vi "xijk_combined_file_save.vi"(8 "error in":errorcluster, 10 "queue in":refnum<queue>, 11 "Settings":T1={"search parameters"={"Paths"={"Path: Excitation filters"=path "", "Path: Dicroic filters"=path "", "Path: Emission filters"=path "", "Path reget"=path ""}, "table excitation"=[], "table dicroics"=[], "table emission"=[], "Integers"={"Select result number"=1}, "boolean selector array"=[], "table for calculation automagic"=[]}, "output cluster"={"Booleans"={"Unknown detector"=FALSE, "Dual band filters"=FALSE, "Dual emission by cubes"=FALSE, "FRET"=FALSE}, "Integers"={"Light source"=0, "Number of fluorophores"=0, "Wavelength of laser (nm) 1"=0, "Broadness of laser (nm) 1"=0.0, "Wavelength of laser (nm) 2"=0, "Broadness of laser (nm) 2"=0.0, "Template"=1}, "Doubles"={"Molar extinction 1"=1.0, "Molar extinction 2"=1.0, "Quantum efficiency 1"=1.0, "Quantum efficiency 2"=1.0}}, "output cluster 2"={"Excitation filter 1"=path "", "Dichroic filter 1"=path "", "Emission filter 1"=path "", "Excitation filter 2"=path "", "Dichroic filter 2"=path "", "Emission filter 2"=path "", "Extra em filter 1"=path "", "Extra em filter 2"=path "", "Light source file"=path "", "Fluorophore absorption 1"=path "", "Fluorophore emission 1"=path "", "Fluorophore absorption 2"=path "", "Fluorophore emission 2"=path "", "Detector"=path ""}, "cluster de sortie"={"Excitation filter_x"=[], "Excitation filter_y"=[], "Dichroic filter_x"=[], "Dichroic filter_y"=[], "Emission filter_x"=[], "Emission filter_y"=[], "Excitation filter_x 2"=[], "Excitation filter_y 2"=[], "Dichroic filter_x 2"=[], "Dichroic filter_y 2"=[], "Emission filter_x 2"=[], "Emission filter_y 2"=[], "Extra em filter_x 1"=[], "Extra em filter_y 1"=[], "Extra em filter_x 1"=[], "Extra em filter_y 2"=[], "Light source_x"=[], "Light source_y"=[], "Detector_x"=[], "Detector_y"=[], "Fluorophore absorption_x"=[], "Fluorophore absorption_y"=[], "Fluorophore emission_x"=[], "Fluorophore emission_y"=[], "Fluorophore absorption_x 2"=[], "Fluorophore absorption_y 2"=[], "Fluorophore emission_x 2"=[], "Fluorophore emission_y 2"=[], "laser_x"=[], "laser_y"=[], "laser_x 2"=[], "laser_y 2"=[], "quantum efficiency factor 1"=0.0, "quantum efficiency factor 2"=0.0, "lamp scaling factor"=0.0}, "Xijk output cluster"={"Xijk 111"=0.0, "Xijk 112"=0.0, "Xijk 121"=0.0, "Xijk 122"=0.0, "Xijk 211"=0.0, "Xijk 212"=0.0, "Xijk 221"=0.0, "Xijk 222"=0.0, "Eijk 111"=0.0, "Eijk 112"=0.0, "Eijk 121"=0.0, "Eijk 122"=0.0, "Eijk 211"=0.0, "Eijk 212"=0.0, "Eijk 221"=0.0, "Eijk 222"=0.0}, "GUI configuration"={"axes in"={"min x-axis excitation"=300, "max x-axis excitation"=800, "min x-axis emission"=300, "max x-axis emission"=800, "precision of results"=2}, "plot colors in"={"Lanscape Portrait"=FALSE, "Plot logarithmic"=FALSE, "Ex/Em filters double"=FALSE, "Line colors"=[16734569, 56375, 16711916, 5896447, 16448250, 56375]}}, "references"={"Excitation filter 1 ref"=refnum, "Dichroic filter 1 ref"=refnum, "Emission filter 1 ref"=refnum, "Excitation filter 2 ref"=refnum, "Dichroic filter 2 ref"=refnum, "Emission filter 2 ref"=refnum, "Extra em filter 1 ref"=refnum, "Extra em filter 2 ref"=refnum, "Light source file ref"=refnum, "Fluorophore absorption 1 ref"=refnum, "Fluorophore emission 1 ref"=refnum, "Fluorophore absorption 2 ref"=refnum, "Fluorophore emission 2 ref"=refnum, "Detector ref"=refnum}} {"GUI configuration"."axes in"."precision of results" max=8 step=1}) -> (0 "error out":errorcluster, 2 "queue out":refnum<queue>, 3 "Settings out":T1 {"GUI configuration"."axes in"."precision of results" max=8 step=1})   [LabVIEW 2009, in "xijk_combined_file.lvlib"]
uses:
  xijk_combined_file.lvlib
  Type Def/event.ctl
  Type Def/settings.ctl
  Type Def/search_parameters.ctl
  Type Def/spectra_parameters.ctl
  Type Def/filepath.ctl
  Type Def/spectrum_table_control.ctl
  Type Def/xijk_cluster.ctl
  Type Def/configuration_cluster.ctl
  Type Def/axis_parameters.ctl
  Type Def/color_parameters.ctl
  Type Def/control_references_cluster.ctl
panel:
  # "Dichroic"
  # "Ex/Em filter"
  # "Fluorophore 1"
  # "Fluorophore 2"
  # "Laser /\nextra Em filter"
  # "Dichroic"
  # "Ex/Em filter"
  # "Fluorophore 1"
  # "Fluorophore 2"
  # "Laser /\nextra Em filter"
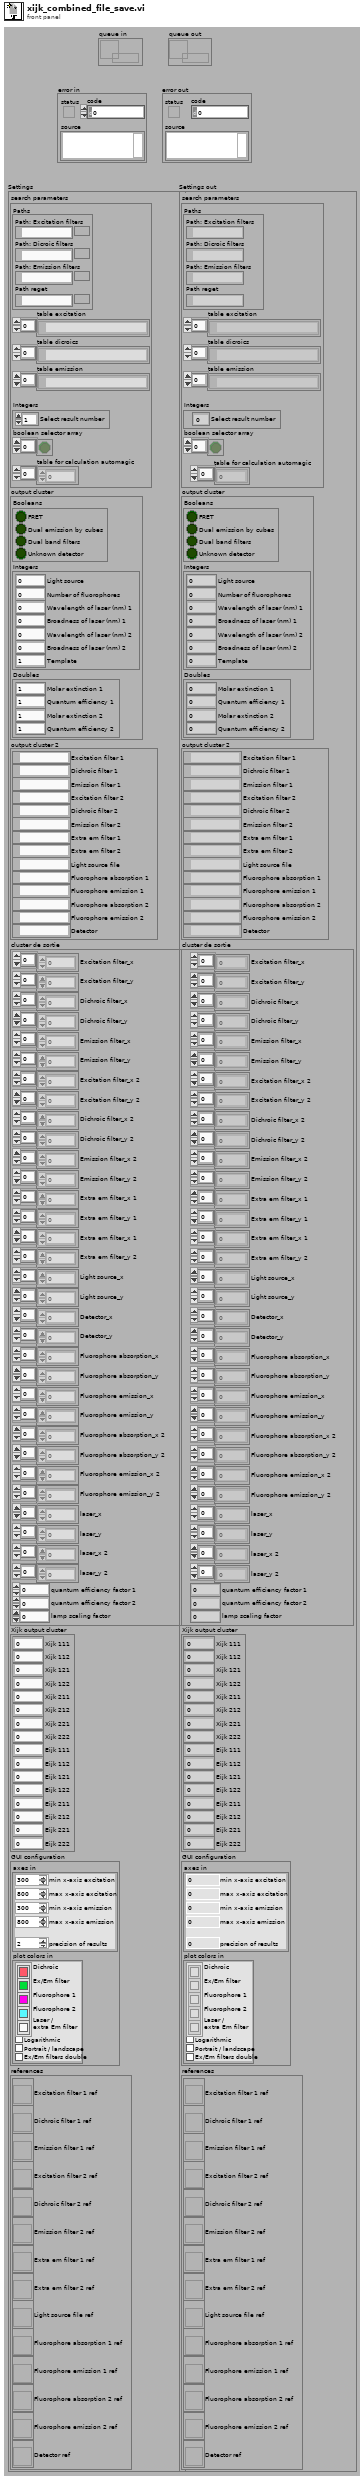
[diagram p1: front panel]
types:
  T1 = typedef "settings.ctl" = cluster{"search parameters":T2, "output cluster":T3, "output cluster 2":T4, "cluster de sortie":T5, "Xijk output cluster":T6, "GUI configuration":T7, "references":T10}
  T2 = typedef "search_parameters.ctl" = cluster{"Paths":cluster{"Path: Excitation filters":path, "Path: Dicroic filters":path, "Path: Emission filters":path, "Path reget":path}, "table excitation":path[], "table dicroics":path[], "table emission":path[], "Integers":cluster{"Select result number":u32}, "boolean selector array":bool[], "table for calculation automagic":i32[]}
  T3 = typedef "spectra_parameters.ctl" = cluster{"Booleans":cluster{"Unknown detector":bool, "Dual band filters":bool, "Dual emission by cubes":bool, "FRET":bool}, "Integers":cluster{"Light source":u16, "Number of fluorophores":u16, "Wavelength of laser (nm) 1":u16, "Broadness of laser (nm) 1":sgl, "Wavelength of laser (nm) 2":u16, "Broadness of laser (nm) 2":sgl, "Template":u16}, "Doubles":cluster{"Molar extinction 1":sgl, "Molar extinction 2":sgl, "Quantum efficiency 1":sgl, "Quantum efficiency 2":sgl}}
  T4 = typedef "filepath.ctl" = cluster{"Excitation filter 1":path, "Dichroic filter 1":path, "Emission filter 1":path, "Excitation filter 2":path, "Dichroic filter 2":path, "Emission filter 2":path, "Extra em filter 1":path, "Extra em filter 2":path, "Light source file":path, "Fluorophore absorption 1":path, "Fluorophore emission 1":path, "Fluorophore absorption 2":path, "Fluorophore emission 2":path, "Detector":path}
  T5 = typedef "spectrum_table_control.ctl" = cluster{"Excitation filter_x":i16[], "Excitation filter_y":sgl[], "Dichroic filter_x":i16[], "Dichroic filter_y":sgl[], "Emission filter_x":i16[], "Emission filter_y":sgl[], "Excitation filter_x 2":i16[], "Excitation filter_y 2":sgl[], "Dichroic filter_x 2":i16[], "Dichroic filter_y 2":sgl[], "Emission filter_x 2":i16[], "Emission filter_y 2":sgl[], "Extra em filter_x 1":i16[], "Extra em filter_y 1":sgl[], "Extra em filter_x 1":i16[], "Extra em filter_y 2":sgl[], "Light source_x":i16[], "Light source_y":sgl[], "Detector_x":i16[], "Detector_y":sgl[], "Fluorophore absorption_x":i16[], "Fluorophore absorption_y":sgl[], "Fluorophore emission_x":i16[], "Fluorophore emission_y":sgl[], "Fluorophore absorption_x 2":i16[], "Fluorophore absorption_y 2":sgl[], "Fluorophore emission_x 2":i16[], "Fluorophore emission_y 2":sgl[], "laser_x":i16[], "laser_y":sgl[], "laser_x 2":i16[], "laser_y 2":sgl[], "quantum efficiency factor 1":sgl, "quantum efficiency factor 2":sgl, "lamp scaling factor":sgl}
  T6 = typedef "xijk_cluster.ctl" = cluster{"Xijk 111":sgl, "Xijk 112":sgl, "Xijk 121":sgl, "Xijk 122":sgl, "Xijk 211":sgl, "Xijk 212":sgl, "Xijk 221":sgl, "Xijk 222":sgl, "Eijk 111":sgl, "Eijk 112":sgl, "Eijk 121":sgl, "Eijk 122":sgl, "Eijk 211":sgl, "Eijk 212":sgl, "Eijk 221":sgl, "Eijk 222":sgl}
  T7 = typedef "configuration_cluster.ctl" = cluster{"axes in":T8, "plot colors in":T9}
  T8 = typedef "axis_parameters.ctl" = cluster{"min x-axis excitation":u16, "max x-axis excitation":u16, "min x-axis emission":u16, "max x-axis emission":u16, "precision of results":u8}
  T9 = typedef "color_parameters.ctl" = cluster{"Lanscape Portrait":bool, "Plot logarithmic":bool, "Ex/Em filters double":bool, "Line colors":u32[]}
  T10 = typedef "control_references_cluster.ctl" = cluster{"Excitation filter 1 ref":refnum<vi>, "Dichroic filter 1 ref":refnum<vi>, "Emission filter 1 ref":refnum<vi>, "Excitation filter 2 ref":refnum<vi>, "Dichroic filter 2 ref":refnum<vi>, "Emission filter 2 ref":refnum<vi>, "Extra em filter 1 ref":refnum<vi>, "Extra em filter 2 ref":refnum<vi>, "Light source file ref":refnum<vi>, "Fluorophore absorption 1 ref":refnum<vi>, "Fluorophore emission 1 ref":refnum<vi>, "Fluorophore absorption 2 ref":refnum<vi>, "Fluorophore emission 2 ref":refnum<vi>, "Detector ref":refnum<vi>}
  T11 = typedef "event.ctl" = enum16{"Initialise parameters", "Initialise paths", "Execute", "Hide detector", "Light source selection", "Get example list", "Set Example", "Change portrait / landscape", "Dual band cube", "Save to file", "Load from file", "Set filepaths to boxes", "1 or 2 fluorophore selection", "Update configurations", "Update template", "Set to personal template", "Calculate other values", "Update filter names", "Shutdown", "Shutdown - hard exit", "Search in filters - set parameters", "Search in filters - search", "Search in filters - get xijk", "Search in filters - reget", "Optimize - Sort table", "Get path from search", "Calculate Xijk", "Get spectra from files", "Create graphs", "Reset variables", "Help - open", "Help - close", "Help - next", "Help - previous", "Help - select menu", "Export data"}
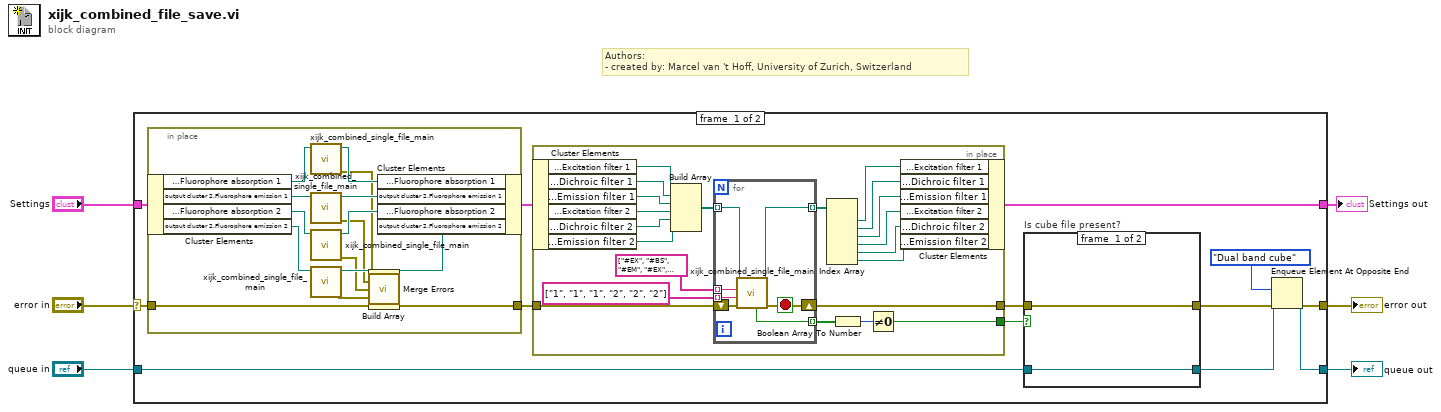
[diagram p0: block diagram]
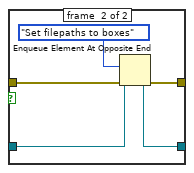
[diagram p2: hidden frame]
diagram:
  # "Authors: \n- created by: Marcel van 't Hoff, University of Zurich, Switzerland"
  n1 = case shown="No Error" "error in" {
    selector: "error in" -> [w10 w72]
    tunnel: [w16 w72] -> w6
    tunnel: "Settings" -> [w11 w71]
    tunnel: [w7 w71] -> w1
    tunnel: [w13 w70] -> w4
    tunnel: "queue in" -> [w18 w70]
    frame #0 {
      n2 = in-place {
        in-place-border: [w50] -> w9
        in-place-border: w10 -> [w49]
        n3 = in-place-cluster #1(w11) -> ("output cluster 2.Fluorophore absorption 1"=w62:path, "output cluster 2.Fluorophore emission 1"=w60:path, "output cluster 2.Fluorophore absorption 2"=w56:path, "output cluster 2.Fluorophore emission 2"=w58:path)
        n4 = call "xijk_combined_single_file_main.vi"("file path in"=w62) -> ("error out"=w51:errorcluster, "file path out"=w61:path)  [unwired: 8 in, 1 out]
        n5 = call "xijk_combined_single_file_main.vi"("file path in"=w60) -> ("error out"=w52:errorcluster, "file path out"=w59:path)  [unwired: 8 in, 1 out]
        n6 = call "xijk_combined_single_file_main.vi"("file path in"=w56) -> ("error out"=w53:errorcluster, "file path out"=w55:path)  [unwired: 8 in, 1 out]
        n7 = call "xijk_combined_single_file_main.vi"("file path in"=w58) -> ("error out"=w54:errorcluster, "file path out"=w57:path)  [unwired: 8 in, 1 out]
        n8 = Build Array(w51, w52, w53, w54, w49) -> (w48:errorcluster[])
        n9 = call <vilib>:"Merge Errors.vi"("error array in"=w48) -> ("error out"=w50:errorcluster)  [unwired: 6 in]
        n10 = in-place-cluster #1("output cluster 2.Fluorophore absorption 1"=w61, "output cluster 2.Fluorophore emission 1"=w59, "output cluster 2.Fluorophore absorption 2"=w55, "output cluster 2.Fluorophore emission 2"=w57) -> (w8:T1)
      }
      n11 = in-place {
        in-place-border: [w34] -> w19
        in-place-border: [w33] -> w12
        in-place-border: w9 -> [w32]
        n12 = in-place-cluster #2(w8) -> ("output cluster 2.Excitation filter 1"=w31:path, "output cluster 2.Dichroic filter 1"=w30:path, "output cluster 2.Emission filter 1"=w29:path, "output cluster 2.Excitation filter 2"=w28:path, "output cluster 2.Dichroic filter 2"=w27:path, "output cluster 2.Emission filter 2"=w26:path)
        n13 = Build Array(w31, w30, w29, w28, w27, w26) -> (w40:path[])
        n14 = for {
          tunnel: w40 -> [w47] mode=indexing
          tunnel: string[] ["#EX", "#BS", "#EM", "#EX", "#BS", "#EM"] -> [w46] mode=indexing
          tunnel: string[] ["1", "1", "1", "2", "2", "2"] -> [w45] mode=indexing
          tunnel: [w43] -> w37 mode=indexing
          tunnel: [w42] -> w36 mode=indexing
          shift-right: [w41] -> w33
          shift-left: w32 -> [w44]
          stop <- w41 stop-if-true
          n15 = call "xijk_combined_single_file_main.vi"("error in (no error)"=w44, "channel"=w45, "element"=w46, "file path in"=w47) -> ("error out"=w41:errorcluster, "file path out"=w43:path, "cube file present?"=w42:bool)  [unwired: 5 in]
        }
        n16 = Index Array(array=w37) -> (element #1=w25:path, element #2=w24:path, element #3=w23:path, element #4=w22:path, element #5=w21:path, element #6=w20:path)  [unwired: 6 in]
        n17 = Boolean Array To Number(Boolean array=w36) -> (number=w35:u32)
        n18 = Not Equal To 0?(x=w35) -> (x != 0?=w34:bool)
        n19 = in-place-cluster #2("output cluster 2.Excitation filter 1"=w25, "output cluster 2.Dichroic filter 1"=w24, "output cluster 2.Emission filter 1"=w23, "output cluster 2.Excitation filter 2"=w22, "output cluster 2.Dichroic filter 2"=w21, "output cluster 2.Emission filter 2"=w20) -> (w7:T1)
      }
      n20 = case "Is cube file present?" shown="True" w19 {
        tunnel: w12 -> [w64 w69]
        tunnel: [w64 w68] -> w17
        tunnel: w18 -> [w63 w67]
        tunnel: [w63 w66] -> w14
        frame #0 {
        }
        frame #1 {
          n21 = Enqueue Element At Opposite End(queue=w67, element=event."Set filepaths to boxes", error in (no error)=w69) -> (queue out=w66:refnum<queue>, error out=w68:errorcluster)  [unwired: 1 in, 1 out]
        }
      }
      n22 = Enqueue Element At Opposite End(queue=w14, element=event."Dual band cube", error in (no error)=w17) -> (queue out=w13:refnum<queue>, error out=w16:errorcluster)  [unwired: 1 in, 1 out]
    }
    frame #1 {
    }
  }
  "error out" <- w6
  "queue out" <- w4
  "Settings out" <- w1
